vi "Test Simple Connection.vi"() -> ()   [LabVIEW 2013]
uses:
  <vilib>/LabVIEW Open Source Project/MQTT Control Packets/Control Packets/CONNECT/CONNECT.lvclass
  <vilib>/LabVIEW Open Source Project/MQTT Control Packets/Control Packets/CONNACK/Connect Return Code -- enum.ctl
  <vilib>/LabVIEW Open Source Project/MQTT Connection/MQTT_Connection/Connection/Connection.lvclass
  <vilib>/LabVIEW Open Source Project/MQTT Control Packets/Control Packets/PUBLISH/PUBLISH.lvclass
  <vilib>/LabVIEW Open Source Project/MQTT Control Packets/Control Packets/ControlPacket/ControlPacket.lvclass
  <vilib>/LabVIEW Open Source Project/MQTT Control Packets/Control Packets/CONNACK/CONNACK.lvclass
  <vilib>/LabVIEW Open Source Project/MQTT Control Packets/Control Packets/ControlPacket/ControlPacket.lvclass/ControlPacket.ctl
  <vilib>/LabVIEW Open Source Project/MQTT Control Packets/Control Packets/DISCONNECT/DISCONNECT.lvclass
  <vilib>/LabVIEW Open Source Project/MQTT Control Packets/Control Packets/MQTT_311/MQTTVersion.lvclass
  <vilib>/LabVIEW Open Source Project/MQTT TCP Connection/MQTT_TCP/Connection/TCPConnection.lvclass
  <vilib>/LabVIEW Open Source Project/MQTT LocalQueue Connection/MQTT_LocalQueue/Connection/LocalQueueConnection.lvclass
  <vilib>/LabVIEW Open Source Project/MQTT Websockets Connection/MQTT_Websockets/Connection/WebsocketsConnection.lvclass
panel:
  in  "Channel Under Test":T1(ring)
  in  "Range (max)":dbl=1.0
  out "randomNumber":dbl
  out "Topic":string
  out "connected":bool
  in  "Connect to Server":bool
  out "client":errorcluster
  out "server":errorcluster
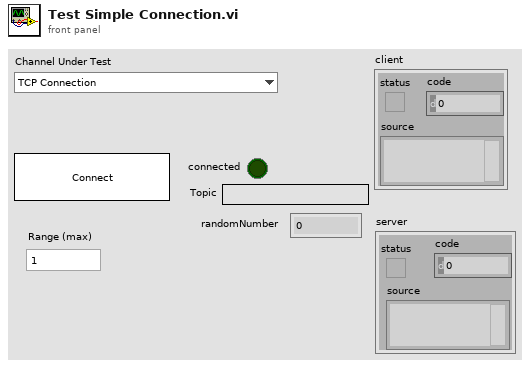
[diagram p1: front panel]
types:
  T1 = enum16{"TCP Connection", "Local Queue Connection", "Websockets"}
  T2 = cluster{"Packet":refnum<class "ControlPacket.lvclass">, "Direction":enum16{"In", "Out"}}
  T3 = cluster{"connected":refnum<user-event>, "Incoming Message":refnum<user-event>}
  T4 = cluster{"Connection":refnum<class "Connection.lvclass">, "Public Events":cluster{"connected":refnum<user-event>, "Incoming Message":refnum<user-event>}, "Payload":refnum<queue>}
  T5 = typedef "MQTT_Control_Packets.lvlib/CONNACK.lvclass/Connect Return Code -- enum.ctl" = enum16{"Connection accepted", "Unacceptable protocol version", "Identifier Rejected", "Server Unavailable", "Bad Username or Password", "Not Authorized"}
  T6 = enum16{"Standard", "Buffered", "CRLF", "Immediate"}
  T7 = typedef "MQTT_Control_Packets.lvlib/ControlPacket.lvclass/Control Packet Type -- enum.ctl" = enum16{"Reserved", "CONNECT", "CONNACK", "PUBLISH", "PUBACK", "PUBREC", "PUBREL", "PUBCOMP", "SUBSCRIBE", "SUBACK", "UNSUBSCRIBE", "UNSUBACK", "PINGREQ", "PINGRESP", "DISCONNECT", "AUTH"}
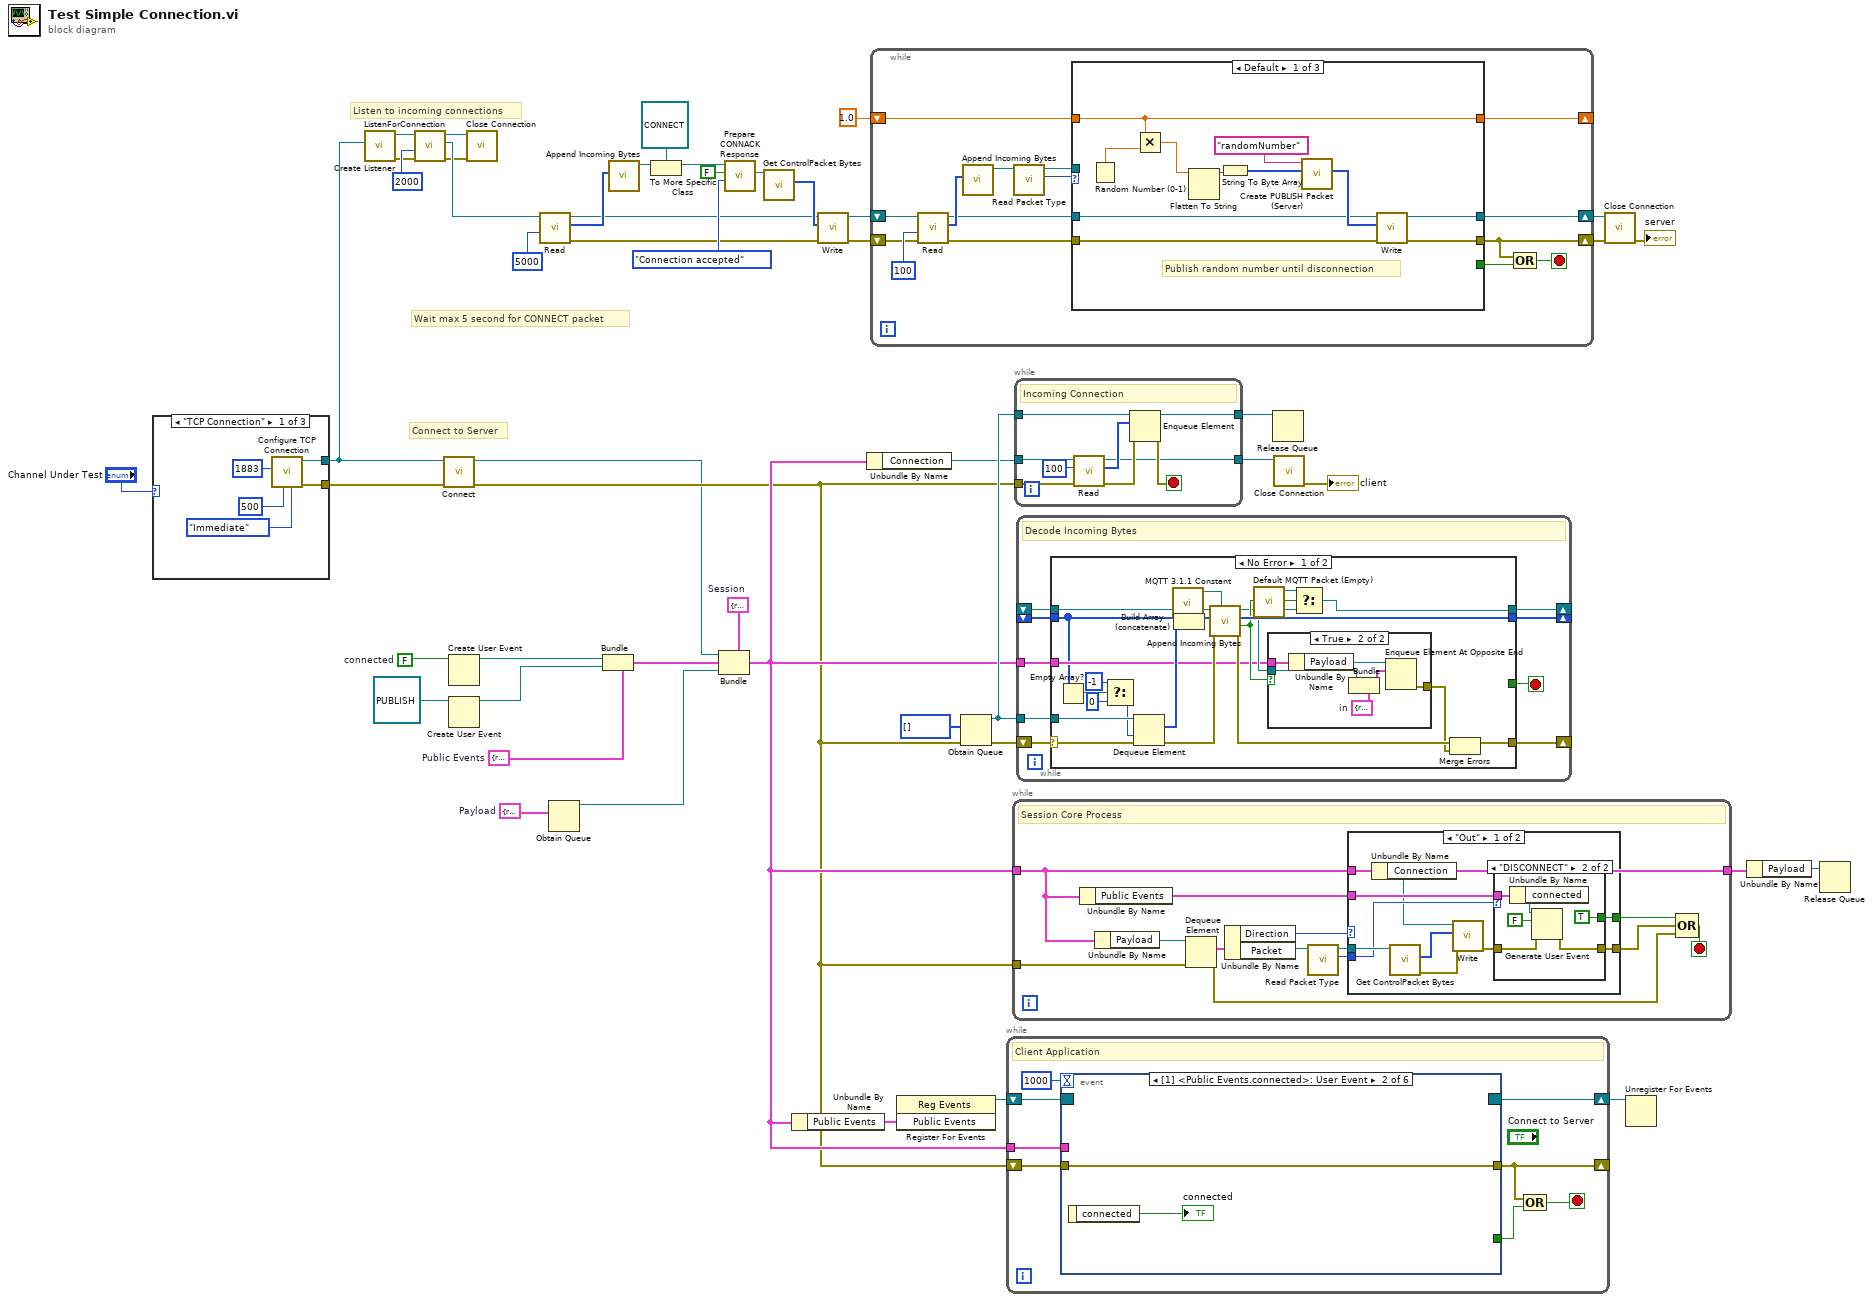
[diagram p0: block diagram]
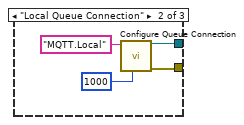
[diagram p2: hidden frame]
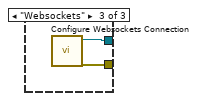
[diagram p3: hidden frame]
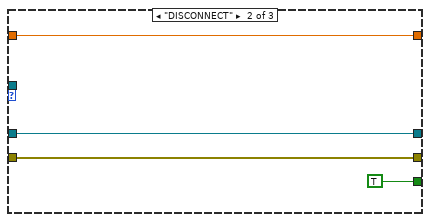
[diagram p4: hidden frame]
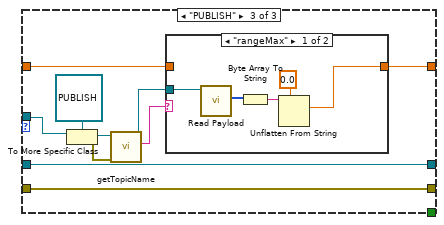
[diagram p5: hidden frame]
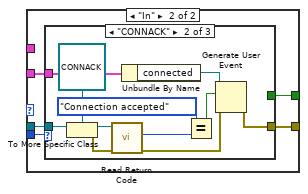
[diagram p8: hidden frame]
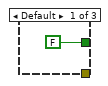
[diagram p9: hidden frame]
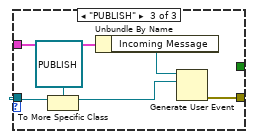
[diagram p10: hidden frame]
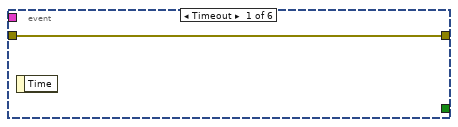
[diagram p11: hidden frame]
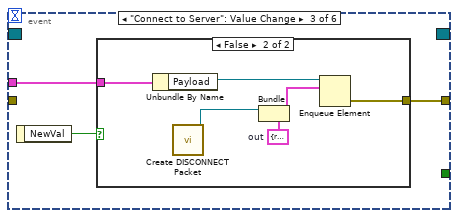
[diagram p12: hidden frame]
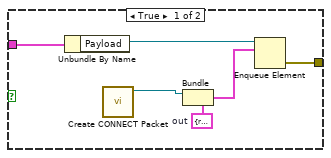
[diagram p13: hidden frame]
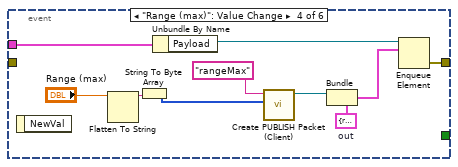
[diagram p14: hidden frame]
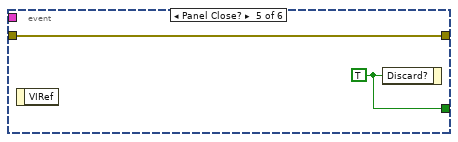
[diagram p15: hidden frame]
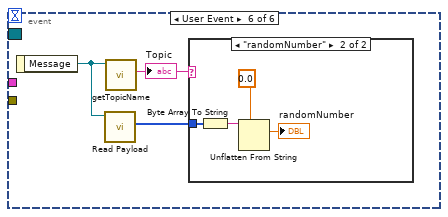
[diagram p16: hidden frame]
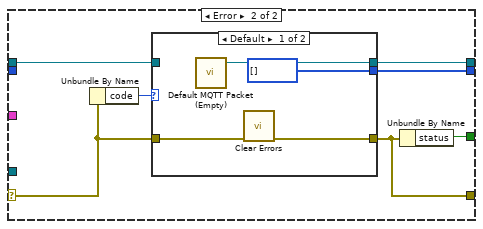
[diagram p19: hidden frame]
diagram:
  w21 = T2 {"Packet"=refnum, "Direction"=enum."In"}  # Payload
  w34 = T3 {"connected"=refnum, "Incoming Message"=refnum}  # Public Events
  w35 = FALSE  # connected
  w37 = T4 {"Connection"=refnum, "Public Events"={"connected"=refnum, "Incoming Message"=refnum}, "Payload"=refnum}  # Session
  # "Connect to Server"
  # "Listen to incoming connections"
  # "Wait max 5 second for CONNECT packet"
  n1 = case shown="\"TCP Connection\"" "Channel Under Test" {
    tunnel: [w52 w57 w61] -> w9
    tunnel: [w51 w58 w60] -> w2
    frame "TCP Connection" {
      n2 = call <vilib>:"Configure TCP Connection.vi"("Read Mode (Immediate)"=T6."Immediate" ("mode (standard)"), "timeout (5000ms)"=500 ("timeout (100ms)"), "remote port (80)"=u16 1883) -> ("error out"=w52:errorcluster, "TCPConnection"=w51:refnum<class "TCPConnection.lvclass">)  [unwired: 7 in]
    }
    frame "Local Queue Connection" {
      n3 = call <vilib>:"Configure Queue Connection.vi"("timeout (500 ms)"=1000 ("timeout (100ms)"), "Queue Name"="MQTT.Local") -> ("error out"=w57:errorcluster, "LocalQueueConnection"=w58:refnum<class "LocalQueueConnection.lvclass">)  [unwired: 8 in]
    }
    frame "Websockets" {
      n4 = call <vilib>:"Configure Websockets Connection.vi"() -> ("error out"=w61:errorcluster, "WSConnection"=w60:refnum<class "WebsocketsConnection.lvclass">)  [unwired: 10 in]
    }
  }
  n5 = call <vilib>:"Create Listener.vi"("Connection Configuration"=w2) -> ("error out"=w4:errorcluster, "Listener"=w8:refnum<class "Connection.lvclass">)  [unwired: 9 in]
  n6 = call <vilib>:"ListenForConnection.vi"("error in (no error)"=w4, "timeout (2000 ms)"=2000 ("bytes to read (100)"), "Listener"=w8) -> ("error out"=w3:errorcluster, "Connection"=w5:refnum<class "Connection.lvclass">, "Listener out"=w6:refnum<class "Connection.lvclass">)  [unwired: 5 in, 1 out]
  n7 = call <vilib>:"Connect.vi"("error in (no error)"=w9, "Connection in"=w2) -> ("error out"=w11:errorcluster, "Connection out"=w10:refnum<class "Connection.lvclass">)  [unwired: 8 in]
  n8 = Create User Event(user event datatype=w35) -> (user event=w36:refnum<user-event>)  [unwired: 1 in, 1 out]
  n9 = Create User Event(user event datatype=refnum<class "PUBLISH.lvclass"> refnum ("Message")) -> (user event=w26:refnum<user-event>)  [unwired: 1 in, 1 out]
  n10 = call <vilib>:"Close Connection.vi"("error in (no error)"=w3, "Connection in"=w6) -> ()  [unwired: 8 in, 2 out]
  n11 = call <vilib>:"Read.vi"("timeout (2000 ms)"=5000 ("bytes to read (100)"), "TCPConnection in"=w5) -> ("error out"=w14:errorcluster, "Bytes"=w13:u8[], "TCPConnection out"=w12:refnum<class "Connection.lvclass">)  [unwired: 5 in, 2 out]
  n12 = Obtain Queue(element data type=w21) -> (queue out=w19:refnum<queue>)  [unwired: 4 in, 2 out]
  n13 = Bundle(cluster=w34, "connected"=w36, "Incoming Message"=w26) -> (w20:T3)
  n14 = call <vilib>:"Append Incoming Bytes.vi"("Incoming Packets"=w13) -> ("ControlPacket"=w50:refnum<class "ControlPacket.lvclass">)  [unwired: 7 in, 3 out]
  n15 = To More Specific Class(target class=refnum<class "CONNECT.lvclass"> refnum ("CONNECT in"), reference=w50) -> (specific class reference=w49:refnum<class "CONNECT.lvclass">)  [unwired: 1 in, 1 out]
  n16 = Bundle(cluster=w37, "Connection"=w10, "Public Events"=w20, "Payload"=w19) -> (w17:T4)
  n17 = call-dynamic "Prepare CONNACK Response.vi"("Return Code"=Connect_Return_Code_--_enum."Connection accepted", "Session Present"=FALSE, "CONNECT in"=w49) -> ("CONNACK response"=w46:refnum<class "CONNACK.lvclass">)  [unwired: 5 in, 3 out]
  n18 = call <vilib>:"Get ControlPacket Bytes.vi"("ControlPacket"=w46) -> ("Bytes Stream"=w47:u8[])  [unwired: 7 in, 3 out]
  n19 = Unbundle By Name(w17) -> ("Public Events"=w33:T3)
  n20 = call <vilib>:"Write.vi"("error in (no error)"=w14, "Bytes"=w47, "Connection in"=w12) -> ("error out"=w24:errorcluster, "Connection"=w25:refnum<class "Connection.lvclass">)  [unwired: 7 in]
  n21 = Unbundle By Name(w17) -> ("Connection"=w16:refnum<class "Connection.lvclass">)
  n22 = while {
    shift-right: [w68] -> w23
    shift-left: w25 -> [w73]
    shift-right: [w65] -> w22
    shift-left: w24 -> [w72]
    shift-right: [w63] -> _
    shift-left: 1.0 -> [w64]
    stop <- w66 stop-if-true
    n23 = call <vilib>:"Read.vi"("error in (no error)"=w72, "timeout (2000 ms)"=100 ("bytes to read (100)"), "TCPConnection in"=w73) -> ("error out"=w69:errorcluster, "Bytes"=w76:u8[], "TCPConnection out"=w70:refnum<class "Connection.lvclass">)  [unwired: 4 in, 2 out]
    n24 = call <vilib>:"Append Incoming Bytes.vi"("Incoming Packets"=w76) -> ("ControlPacket"=w75:refnum<class "ControlPacket.lvclass">)  [unwired: 7 in, 3 out]
    n25 = call <vilib>:"Read Packet Type.vi"("ControlPacket in"=w75) -> ("Control Packet Type"=w71:T7, "ControlPacket out"=w62:refnum<class "ControlPacket.lvclass">)  [unwired: 9 in]
    n26 = case shown="Default" w71 {
      tunnel: w70 -> [w83 w91 w101]
      tunnel: w69 -> [w80 w90 w100]
      tunnel: [w82 w91 w101] -> w68
      tunnel: [w81 w90 w100] -> w65
      tunnel: [_ TRUE _] -> w67
      tunnel: w64 -> [w77 w88 w94]
      tunnel: [w77 w88 w93] -> w63
      tunnel: w62 -> [_ _ w98]
      frame Default {
        # "Publish random number until disconnection"
        n27 = Random Number (0-1)() -> (number: 0 to 1=w79:dbl)
        n28 = Multiply(x=w77, y=w79) -> (x*y=w78:dbl)
        n29 = Flatten To String(anything=w78) -> (data string=w85:string)  [unwired: 3 in, 2 out]
        n30 = String To Byte Array(string=w85) -> (unsigned byte array=w86:u8[])
        n31 = call <vilib>:"Create PUBLISH Packet (Server).vi"("Payload"=w86, "Topic Name"="randomNumber") -> ("Bytes Stream"=w87:u8[])  [unwired: 6 in, 3 out]
        n32 = call <vilib>:"Write.vi"("error in (no error)"=w80, "Bytes"=w87, "Connection in"=w83) -> ("error out"=w81:errorcluster, "Connection"=w82:refnum<class "Connection.lvclass">)  [unwired: 7 in]
      }
      frame "DISCONNECT" {
      }
      frame "PUBLISH" {
        n33 = To More Specific Class(target class=refnum<class "PUBLISH.lvclass"> refnum ("event data"), reference=w98) -> (specific class reference=w96:refnum<class "PUBLISH.lvclass">, error out=w97:errorcluster)  [unwired: 1 in]
        n34 = call <vilib>:"getTopicName.vi"("error in (no error)"=w97, "PUBLISH in"=w96) -> ("Topic"=w95:string, "PUBLISH out"=w92:refnum<class "PUBLISH.lvclass">)  [unwired: 7 in, 1 out]
        n35 = case shown="\"rangeMax\"" w95 {
          tunnel: w94 -> [_ w107]
          tunnel: [w102 w107] -> w93
          tunnel: w92 -> [w106 _]
          frame "rangeMax" {
            n36 = call <vilib>:"Read Payload.vi"("ControlPacket in"=w106) -> ("Payload"=w103:u8[])  [unwired: 9 in, 1 out]
            n37 = Byte Array To String(unsigned byte array=w103) -> (string=w104:string)
            n38 = Unflatten From String(type=0.0, binary string=w104) -> (value=w102:dbl)  [unwired: 3 in, 2 out]
          }
          frame Default {
          }
        }
      }
    }
    n39 = Compound Arithmetic op=OR(w65, w67) -> (w66:bool)
  }
  n40 = register-events(w33) -> (reference out=w39:refnum<event-registration>)  [unwired: 2 in, 1 out]
  n41 = Obtain Queue(element data type=u8[] [] ("Remaining Packets"), error in (no error)=w11) -> (queue out=w43:refnum<queue>, error out=w41:errorcluster)  [unwired: 3 in, 1 out]
  n42 = while {
    shift-right: [w113] -> w38
    shift-left: w39 -> [w114]
    shift-right: [w111] -> _
    shift-left: w11 -> [w112]
    tunnel: w17 -> [w109]
    stop <- w110 stop-if-true
    # "Client Application"
    n43 = event shown="[1] <Public Events.connected>: User Event" {
      selector: w114 -> [_ _ _ _ _ _]
      dyn-events: [_ _ _ _ _ _] -> w113
      timeout: 1000 -> [_ _ _ _ _ _]
      tunnel: [_ _ _ _ w145 _] -> w108
      tunnel: [w116 w118 w119 w142 w144 _] -> w111
      tunnel: w112 -> [w116 w118 _ _ w144 _]
      tunnel: w109 -> [_ _ w120 w143 _ _]
      event Timeout {
        n44 = event-data() -> ()  [unwired: 1 in, 1 out]
      }
      event User Event {
        n45 = event-data() -> ("connected"=→"connected":bool)  [unwired: 1 in]
      }
      event "Connect to Server": Value Change {
        n46 = event-data() -> ("NewVal"=w121:bool)  [unwired: 1 in]
        n47 = case shown="False" w121 {
          tunnel: w120 -> [w127 w133]
          tunnel: [w125 w131] -> w119
          frame True {
            w124 = T2 {"Packet"=refnum, "Direction"=enum."Out"}  # out
            n48 = Unbundle By Name(w127) -> ("Payload"=w126:refnum<queue>)
            n49 = call <vilib>:"Create CONNECT Packet.vi"() -> ("CONNECT"=w123:refnum<class "CONNECT.lvclass">)  [unwired: 9 in, 2 out]
            n50 = Bundle(cluster=w124, "Packet"=w123) -> (w122:T2)  [unwired: 1 in]
            n51 = Enqueue Element(queue=w126, element=w122) -> (error out=w125:errorcluster)  [unwired: 2 in, 2 out]
          }
          frame False {
            w128 = T2 {"Packet"=refnum, "Direction"=enum."Out"}  # out
            n52 = Unbundle By Name(w133) -> ("Payload"=w132:refnum<queue>)
            n53 = call <vilib>:"Create DISCONNECT Packet.vi"() -> ("DISCONNECT"=w130:refnum<class "DISCONNECT.lvclass">)  [unwired: 9 in, 2 out]
            n54 = Bundle(cluster=w128, "Packet"=w130) -> (w129:T2)  [unwired: 1 in]
            n55 = Enqueue Element(queue=w132, element=w129) -> (error out=w131:errorcluster)  [unwired: 2 in, 2 out]
          }
        }
      }
      event "Range (max)": Value Change {
        w140 = T2 {"Packet"=refnum, "Direction"=enum."Out"}  # out
        n56 = event-data() -> ()  [unwired: 1 in, 1 out]
        n57 = Flatten To String(anything="Range (max)") -> (data string=w136:string)  [unwired: 3 in, 2 out]
        n58 = String To Byte Array(string=w136) -> (unsigned byte array=w135:u8[])
        n59 = Unbundle By Name(w143) -> ("Payload"=w141:refnum<queue>)
        n60 = call <vilib>:"Create PUBLISH Packet (Client).vi"("Payload"=w135, "Topic Name"="rangeMax") -> ("PUBLISH"=w138:refnum<class "PUBLISH.lvclass">)  [unwired: 6 in, 3 out]
        n61 = Bundle(cluster=w140, "Packet"=w138) -> (w139:T2)  [unwired: 1 in]
        n62 = Enqueue Element(queue=w141, element=w139) -> (error out=w142:errorcluster)  [unwired: 2 in, 2 out]
      }
      event Panel Close? {
        w145 = TRUE ("Discard?")
        n63 = event-data() -> ()  [unwired: 1 in, 1 out]
        n64 = event-data("Discard?"=w145) -> ()  [unwired: 1 in, 1 out]
      }
      event User Event {
        n65 = event-data() -> ("Message"=w148:refnum<class "PUBLISH.lvclass">)  [unwired: 1 in]
        n66 = call <vilib>:"Read Payload.vi"("ControlPacket in"=w148) -> ("Payload"=w146:u8[])  [unwired: 9 in, 1 out]
        n67 = call <vilib>:"getTopicName.vi"("PUBLISH in"=w148) -> ("Topic"=w147:string)  [unwired: 8 in, 2 out]
        "Topic" <- w147
        n68 = case shown="\"randomNumber\"" w147 {
          tunnel: w146 -> [_ w151]
          frame "False", Default {
          }
          frame "randomNumber" {
            n69 = Byte Array To String(unsigned byte array=w151) -> (string=w150:string)
            n70 = Unflatten From String(type=0.0, binary string=w150) -> (value=→"randomNumber":dbl)  [unwired: 3 in, 2 out]
          }
        }
      }
    }
    n71 = Compound Arithmetic op=OR(w111, w108) -> (w110:bool)
  }
  n72 = while {
    tunnel: w17 -> [w154]
    tunnel: [w154] -> w32
    tunnel: w11 -> [w163]
    stop <- w159 stop-if-true
    # "Session Core Process"
    n73 = Unbundle By Name(w154) -> ("Public Events"=w153:T3)
    n74 = Unbundle By Name(w154) -> ("Payload"=w158:refnum<queue>)
    n75 = Dequeue Element(queue=w158, error in (no error)=w163) -> (element=w157:T2, error out=w160:errorcluster)  [unwired: 1 in, 2 out]
    n76 = Unbundle By Name(w157) -> ("Direction"=w155:enum16{"In", "Out"}, "Packet"=w156:refnum<class "ControlPacket.lvclass">)
    n77 = call <vilib>:"Read Packet Type.vi"("ControlPacket in"=w156) -> ("Control Packet Type"=w165:T7, "ControlPacket out"=w164:refnum<class "ControlPacket.lvclass">)  [unwired: 9 in]
    n78 = case shown="\"Out\"" w155 {
      tunnel: w165 -> [w171 w187]
      tunnel: w164 -> [w173 w186]
      tunnel: [w175 w185] -> w162
      tunnel: [w174 w184] -> w161
      tunnel: w154 -> [w172 _]
      tunnel: w153 -> [w170 w183]
      frame "Out" {
        n79 = Unbundle By Name(w172) -> ("Connection"=w169:refnum<class "Connection.lvclass">)
        n80 = call <vilib>:"Get ControlPacket Bytes.vi"("ControlPacket"=w173) -> ("error out"=w167:errorcluster, "Bytes Stream"=w168:u8[])  [unwired: 7 in, 2 out]
        n81 = call <vilib>:"Write.vi"("error in (no error)"=w167, "Bytes"=w168, "Connection in"=w169) -> ("error out"=w166:errorcluster)  [unwired: 7 in, 1 out]
        n82 = case shown="\"DISCONNECT\"" w171 {
          tunnel: [_ TRUE] -> w175
          tunnel: [w176 w180] -> w174
          tunnel: w166 -> [w176 w179]
          tunnel: w170 -> [_ w178]
          frame Default {
          }
          frame "DISCONNECT" {
            n83 = Unbundle By Name(w178) -> ("connected"=w177:refnum<user-event>)
            n84 = Generate User Event(user event=w177, event data cluster=FALSE ("event data"), error in=w179) -> (error out=w180:errorcluster)  [unwired: 1 in, 1 out]
          }
        }
      }
      frame "In" {
        n85 = case shown="\"CONNACK\"" w187 {
          tunnel: w186 -> [_ w199 w204]
          tunnel: [_ w194 w205] -> w184
          tunnel: [FALSE _ _] -> w185
          tunnel: w183 -> [_ w189 w201]
          frame Default {
          }
          frame "CONNACK" {
            n86 = To More Specific Class(target class=refnum<class "CONNACK.lvclass"> refnum ("CONNACK in"), reference=w199) -> (specific class reference=w197:refnum<class "CONNACK.lvclass">, error out=w192:errorcluster)  [unwired: 1 in]
            n87 = call <vilib>:"Read Return Code.vi"("error in (no error)"=w192, "CONNACK in"=w197) -> ("error out"=w193:errorcluster, "Return Code"=w196:T5)  [unwired: 7 in, 1 out]
            n88 = Unbundle By Name(w189) -> ("connected"=w190:refnum<user-event>)
            n89 = Equal?(x=Connect_Return_Code_--_enum."Connection accepted", y=w196) -> (x = y?=w195:bool)
            n90 = Generate User Event(user event=w190, event data cluster=w195, error in=w193) -> (error out=w194:errorcluster)  [unwired: 1 in, 1 out]
          }
          frame "PUBLISH" {
            n91 = To More Specific Class(target class=refnum<class "PUBLISH.lvclass"> refnum ("event data"), reference=w204) -> (specific class reference=w202:refnum<class "PUBLISH.lvclass">)  [unwired: 1 in, 1 out]
            n92 = Unbundle By Name(w201) -> ("Incoming Message"=w200:refnum<user-event>)
            n93 = Generate User Event(user event=w200, event data cluster=w202) -> (error out=w205:errorcluster)  [unwired: 2 in, 1 out]
          }
        }
      }
    }
    n94 = Compound Arithmetic op=OR(w162, w161, w160) -> (w159:bool)
  }
  n95 = while {
    tunnel: w43 -> [w214]
    tunnel: w16 -> [w211]
    tunnel: [w206] -> w40
    tunnel: [w213] -> w30
    tunnel: w11 -> [w209]
    stop <- w212 stop-if-true
    # "Incoming Connection"
    n96 = call <vilib>:"Read.vi"("error in (no error)"=w209, "bytes to read (100)"=100, "TCPConnection in"=w211) -> ("error out"=w208:errorcluster, "Bytes"=w207:u8[], "TCPConnection out"=w206:refnum<class "Connection.lvclass">)  [unwired: 4 in, 2 out]
    n97 = Enqueue Element(queue=w214, element=w207, error in (no error)=w208) -> (queue out=w213:refnum<queue>, error out=w212:errorcluster)  [unwired: 1 in, 1 out]
  }
  n98 = while {
    shift-right: [w221] -> _
    shift-left: _ -> [w220]
    shift-right: [w219] -> _
    shift-left: w41 -> [w218]
    shift-right: [w222] -> _
    shift-left: _ -> [w223]
    tunnel: w17 -> [w215]
    tunnel: w43 -> [w216]
    stop <- w217 stop-if-true
    # "Decode Incoming Bytes"
    n99 = case shown="No Error" w218 {
      selector: w218 -> [w238 w255]
      tunnel: w223 -> [w244 w253]
      tunnel: [w234 w257] -> w222
      tunnel: [w242 w256] -> w221
      tunnel: w220 -> [w225 _]
      tunnel: [w235 w252] -> w219
      tunnel: [_ w251] -> w217
      tunnel: w216 -> [w241 _]
      tunnel: w215 -> [w229 _]
      frame No Error {
        # "No Error"
        n100 = Empty Array?(array=w225) -> (empty?=w228:bool)
        n101 = Select(t=-1 ("timeout in ms (-1)"), s=w228, f=0) -> (s? t:f=w224:i32)
        n102 = Dequeue Element(queue=w241, timeout in ms (-1)=w224, error in (no error)=w238) -> (element=w240:u8[], error out=w237:errorcluster)  [unwired: 2 out]
        n103 = call <vilib>:"MQTT 3.1.1 Constant.vi"() -> ("MQTT 3.1.1"=w243:refnum<class "MQTTVersion.lvclass">)  [unwired: 11 in]
        n104 = Build Array (concatenate)(w225, w240) -> (w239:u8[])
        n105 = call <vilib>:"Append Incoming Bytes.vi"("MQTT Version (3.1.1)"=w243, "error in (no error)"=w237, "Incoming Packets"=w239, "Incomplete ControlPacket"=w244) -> ("error out"=w236:errorcluster, "Complete Packet"=w232:bool, "Remaining Packets"=w242:u8[], "ControlPacket"=w231:refnum<class "ControlPacket.lvclass">)  [unwired: 4 in]
        n106 = call <vilib>:"Default MQTT Packet (Empty).vi"() -> ("No Packet"=w233:refnum<class "ControlPacket.lvclass">)  [unwired: 11 in]
        n107 = case shown="True" w232 {
          tunnel: [_ w250] -> w230
          tunnel: w231 -> [_ w247]
          tunnel: w229 -> [_ w245]
          frame False {
            # "No Packet received"
          }
          frame True {
            w249 = T2 {"Packet"=refnum, "Direction"=enum."In"}  # in
            # "Packet Received"
            n108 = Unbundle By Name(w245) -> ("Payload"=w246:refnum<queue>)
            n109 = Bundle(cluster=w249, "Packet"=w247) -> (w248:T2)  [unwired: 1 in]
            n110 = Enqueue Element At Opposite End(queue=w246, element=w248) -> (error out=w250:errorcluster)  [unwired: 2 in, 2 out]
          }
        }
        n111 = Select(t=w233, s=w232, f=w231) -> (s? t:f=w234:refnum<class "ControlPacket.lvclass">)
        n112 = Merge Errors(w236, w230) -> (w235:errorcluster)
      }
      frame Error {
        # "Handle Error"
        n113 = Unbundle By Name(w255) -> ("code"=w254:i32)
        n114 = case shown="Default" w254 {
          tunnel: [w258 w263] -> w257
          tunnel: w255 -> [w261 w262]
          tunnel: [w260 w262] -> w252
          tunnel: [u8[] [] ("Remaining Packets") _] -> w256
          tunnel: w253 -> [_ w263]
          frame Default {
            # "Malformed Packet"
            n115 = call <vilib>:"Default MQTT Packet (Empty).vi"() -> ("No Packet"=w258:refnum<class "ControlPacket.lvclass">)  [unwired: 11 in]
            n116 = call <vilib>:"Clear Errors.vi"("error in (no error)"=w261) -> ("error out"=w260:errorcluster)  [unwired: 6 in]
          }
          frame 1, 66, 1556 {
          }
        }
        n117 = Unbundle By Name(w252) -> ("status"=w251:bool)
      }
    }
  }
  n118 = Release Queue(queue=w30) -> ()  [unwired: 2 in, 3 out]
  n119 = call <vilib>:"Close Connection.vi"("Connection in"=w40) -> ("error out"=→"client":errorcluster)  [unwired: 9 in, 1 out]
  n120 = call <vilib>:"Close Connection.vi"("error in (no error)"=w22, "Connection in"=w23) -> ("error out"=→"server":errorcluster)  [unwired: 8 in, 1 out]
  n121 = Unregister For Events(event registration refnum=w38) -> ()  [unwired: 1 in, 1 out]
  n122 = Unbundle By Name(w32) -> ("Payload"=w31:refnum<queue>)
  n123 = Release Queue(queue=w31) -> ()  [unwired: 2 in, 3 out]
